vi "Set Bucket Versioning.vi"(4 "Region":T1, 6 "Auth device data":T2, 7 "Versioning Configuration":T3={"Status"=enum."Suspended", "MfaDelete"=enum."Disabled"}, 8 "error in (no error)":errorcluster, 9 "Bucket":string) -> (0 "error out":errorcluster)   [LabVIEW 2015, in "LV Interface for Amazon S3.lvlib"]
doc: "This operation <B>sets the versioning state of an existing bucket</B>. To set the versioning state, you <B>must be the bucket owner</B>."
uses:
  LV Interface for Amazon S3.lvlib
  Typedefs/AMZ_S3_API_VersioningConfiguration.ctl
  Typedefs/AMZ_S3_Versioning Status.ctl
  Typedefs/AMZ_S3_MFA Delete.ctl
  Typedefs/AMZ_S3_Auth Device Data.ctl
  Typedefs/AMZ_S3_LocationConstraint.ctl
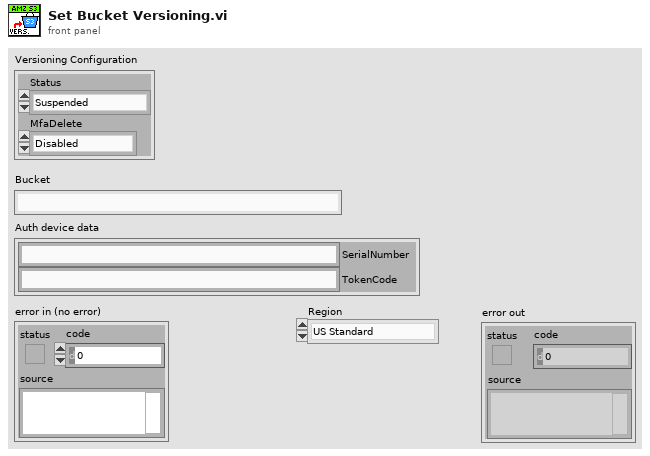
[diagram p1: front panel]
types:
  T1 = typedef "LV Interface for Amazon S3.lvlib/AMZ_S3_LocationConstraint.ctl" = enum16{"US Standard", "us-east-2", "us-west-1", "us-west-2", "ap-northeast-1", "ap-northeast-2", "ap-southeast-1", "ap-southeast-2", "ca-central-1", "eu-central-1", "eu-west-1", "eu-west-2", "sa-east-1"}
  T2 = typedef "LV Interface for Amazon S3.lvlib/AMZ_S3_Auth Device Data.ctl" = cluster{"SerialNumber":string, "TokenCode":string}
  T3 = typedef "LV Interface for Amazon S3.lvlib/AMZ_S3_API_VersioningConfiguration.ctl" = cluster{"Status":T4, "MfaDelete":T5}
  T4 = typedef "LV Interface for Amazon S3.lvlib/AMZ_S3_Versioning Status.ctl" = enum16{"Disabled", "Suspended", "Enabled"}
  T5 = typedef "LV Interface for Amazon S3.lvlib/AMZ_S3_MFA Delete.ctl" = enum16{"Disabled", "Enabled"}
  T6 = typedef "LV Interface for Amazon S3.lvlib/AMZ_S3_HTTP Header-Value pair.ctl" = cluster{"Header":string, "Value":string}
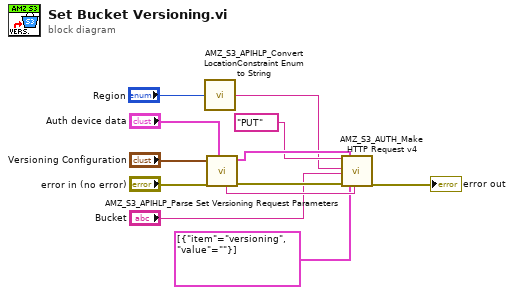
[diagram p0: block diagram]
diagram:
  n1 = call "AMZ_S3_APIHLP_Convert LocationConstraint Enum to String.vi"("Location"="Region") -> ("Location String"=w1:string)  [unwired: 4 in]
  n2 = call "AMZ_S3_APIHLP_Parse Set Versioning Request Parameters.vi"("Auth device data"="Auth device data", "error in (no error)"="error in (no error)", "VersioningConfiguration"="Versioning Configuration") -> ("error out"=w9:errorcluster, "HTTP Headers"=w7:T6[], "PUT Data"=w8:string)  [unwired: 5 in]
  n3 = call "AMZ_S3_AUTH_Make HTTP Request v4.vi"("HTTP-Verb"="PUT", "Region"=w1, "Bucket"="Bucket", "error in"=w9, "request headers"=w7, "request parameters"=cluster{"item":string, "value":string}[] [{"item"="versioning", "value"=""}], "request body"=w8) -> ("error out"=→"error out":errorcluster)  [unwired: 9 in, 3 out]
